vi "CALL_MAIN_2.vi"(10 "Sub Panel":refnum<vi>, 11 "simulazione":bool) -> ()   [LabVIEW 2019]
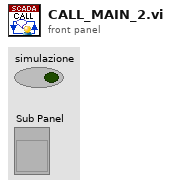
[diagram p1: front panel]
types:
  T1 = enum16{"Left Button", "Center Button", "Right Button", "Window Close"}
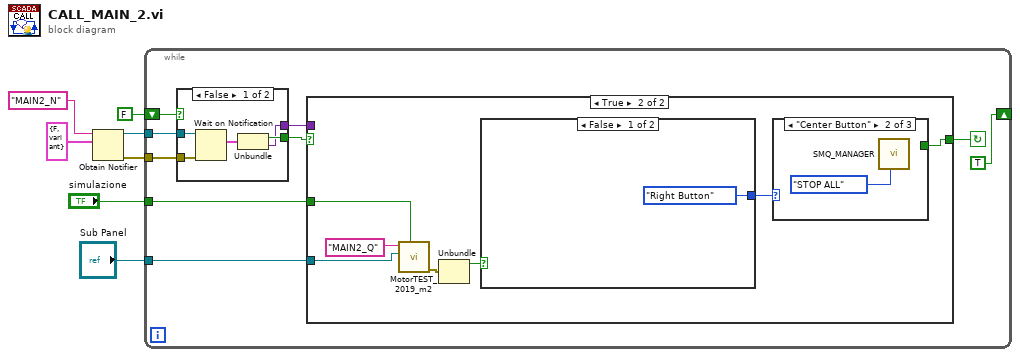
[diagram p0: block diagram]
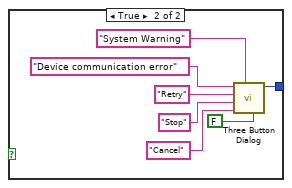
[diagram p4: hidden frame]
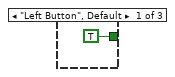
[diagram p5: hidden frame]
diagram:
  n1 = Obtain Notifier(name (unnamed)="MAIN2_N" ("Notifier Name"), notification data type=cluster{"boolean":bool, "variant":variant} {"boolean"=FALSE, "variant"=variant} ("notification")) -> (notifier out=w5:refnum<notifier>, error out=w6:errorcluster)  [unwired: 2 in, 1 out]
  n2 = while {
    tunnel: "simulazione" -> [w15]
    tunnel: w6 -> [w13]
    tunnel: w5 -> [w14]
    shift-right: [TRUE] -> _
    shift-left: FALSE -> [w10]
    tunnel: "Sub Panel" -> [w8]
    stop <- w16 continue-if-true
    n3 = case shown="False" w10 {
      selector: w10 -> [_ w22]
      tunnel: w14 -> [w21 _]
      tunnel: w13 -> [w20 _]
      tunnel: [w18 w22] -> w12
      tunnel: [w17 _] -> w11
      frame False {
        n4 = Wait on Notification(notifier=w21, error in (no error)=w20) -> (notification=w19:cluster{"boolean":bool, "variant":variant})  [unwired: 2 in, 3 out]
        n5 = Unbundle(w19) -> ("boolean"=w18:bool, "variant"=w17:variant)
      }
      frame True {
      }
    }
    n6 = case shown="True" w12 {
      selector: w12 -> [w23 _]
      tunnel: [w23 w28] -> w16
      tunnel: w11 -> [_ _]
      tunnel: w15 -> [_ w25]
      tunnel: w8 -> [_ w24]
      frame False {
      }
      frame True {
        n7 = call "MotorTEST_2019_m2.vi"("simulazione"=w25, "Sub Panel"=w24, "Queue Name"="MAIN2_Q") -> ("error out"=w26:errorcluster)  [unwired: 7 in, 1 out]
        n8 = Unbundle(w26) -> ("status"=w30:bool)  [unwired: 2 out]
        n9 = case shown="False" w30 {
          tunnel: [T1."Right Button" ("Which Button?") w32] -> w29
          frame False {
          }
          frame True {
            n10 = call <vilib>:"Three Button Dialog.vi"("Allow user to close window? (TRUE)"=FALSE, "Window Title (\"\")"="System Warning" ("Window Title (\"\")"), "Right Button Text (\"Cancel\")"="Cancel" ("Right Button Text (\"Cancel\")"), "Center Button Text (\"No\")"="Stop" ("Center Button Text (\"No\")"), "Left Button Text (\"Yes\")"="Retry" ("Left Button Text (\"Yes\")"), "message"="Device communication error") -> ("Which Button?"=w32:T1)  [unwired: 5 in]
          }
        }
        n11 = case shown="\"Center Button\"" w29 {
          tunnel: [TRUE ("Allow user to close window? (TRUE)") _ _] -> w28
          frame "Left Button", Default {
          }
          frame "Center Button" {
            n12 = call <userlib>:"SMQ_MANAGER.vi"("Function"=enum16{"INITIALIZE", "ENQUEUE", "STOP ALL"}."STOP ALL") -> ()  [unwired: 10 in, 1 out]
          }
          frame "Right Button" {
          }
        }
      }
    }
  }
